vi "delete.vi"(8 "error in (no error)":errorcluster, 11 "node ref":refnum<data-value>) -> (0 "error out":errorcluster)   [LabVIEW 2021, in "IDoublyNode.lvclass"]
uses:
  IDoublyNode.lvclass
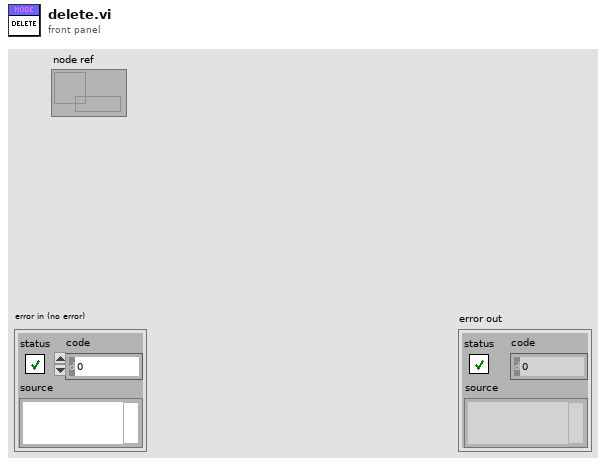
[diagram p1: front panel]
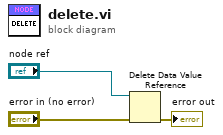
[diagram p0: block diagram]
diagram:
  n1 = Delete Data Value Reference(data value reference="node ref", error in="error in (no error)") -> (error out=→"error out":errorcluster)  [unwired: 1 out]
